vi "sqlread_write.vi"() -> ()   [LabVIEW 2017]
uses:
  <vilib>/addons/database/Connection.llb/DB Tools Open Connec (Path).vi
  <vilib>/addons/database/NI_Database_API.lvlib
panel:
  out "TRUE no barcode Done on station 1":bool
  out "FALSE healty":bool
  out "TRUE Duplication on Station 2":bool
  out "data":string[][](array[string])
  out "error out":errorcluster
  in  "error in (no error)":errorcluster
  # "testing vi"
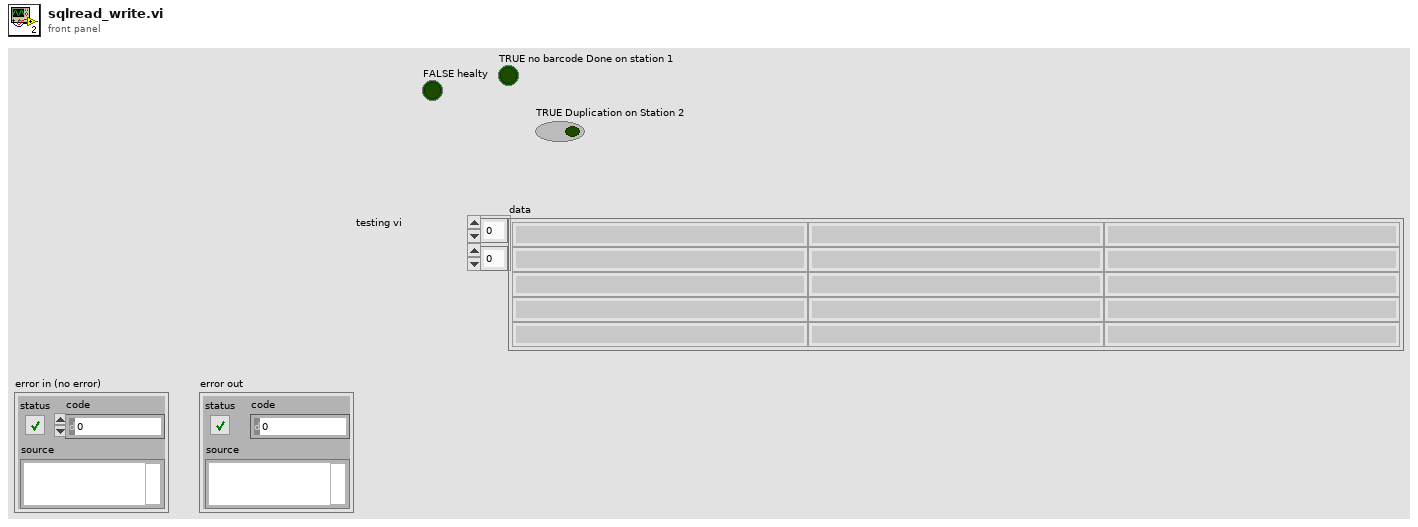
[diagram p1: front panel]
types:
  T1 = typedef "NI_Database_API.lvlib/Conn ObjectReference.ctl" = refnum<k1>
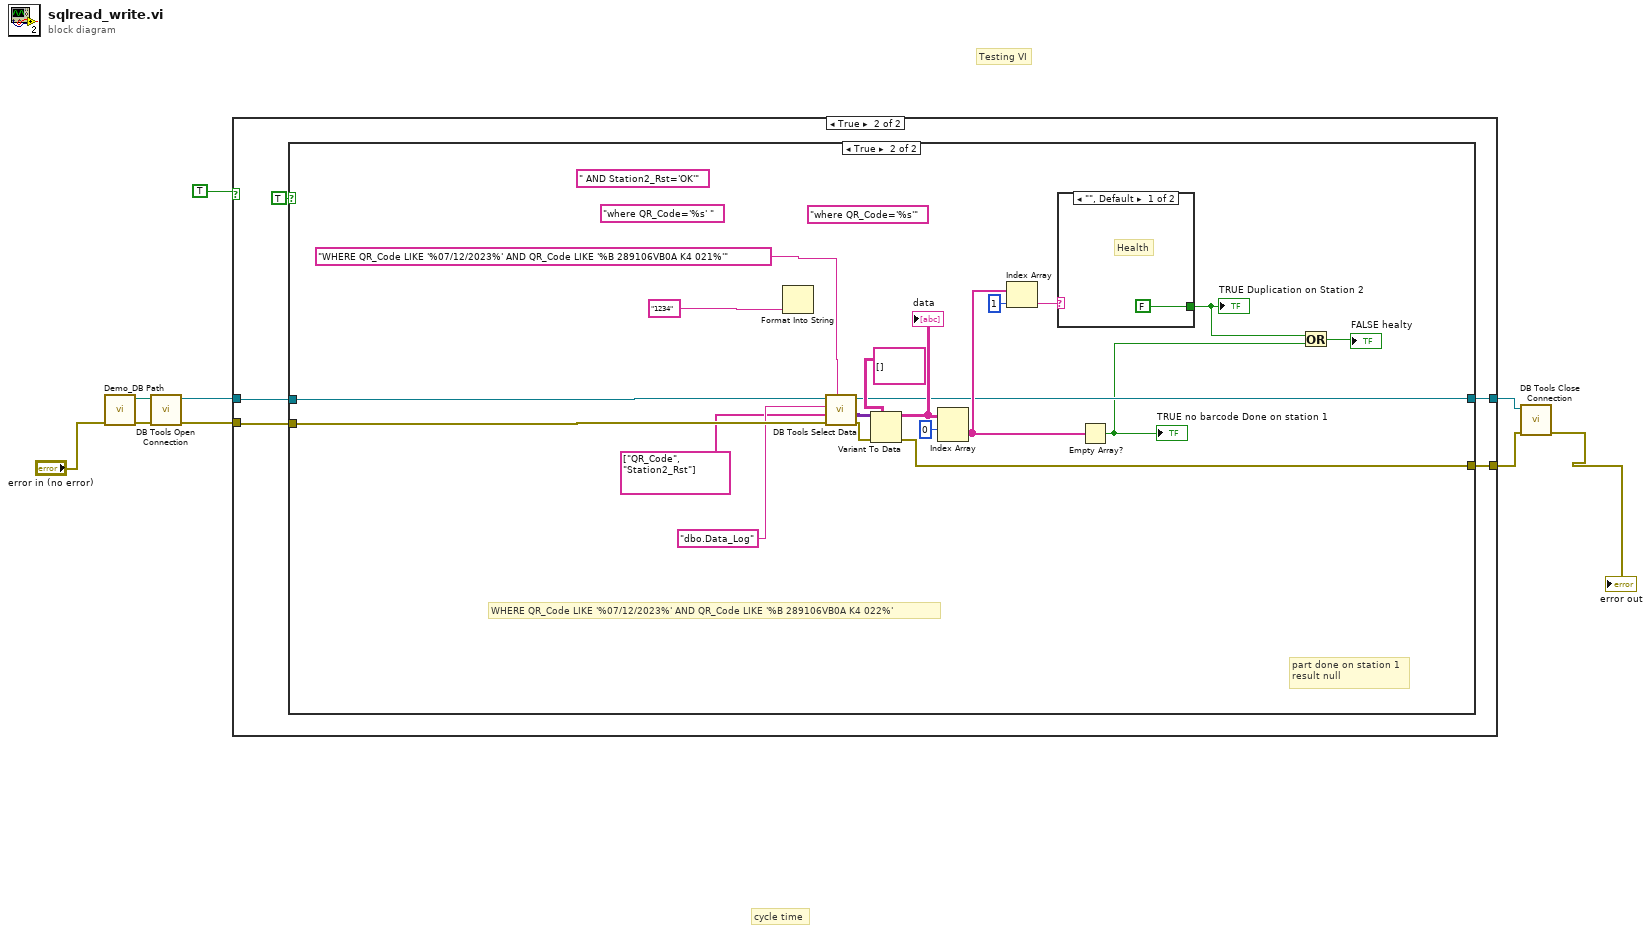
[diagram p0: block diagram]
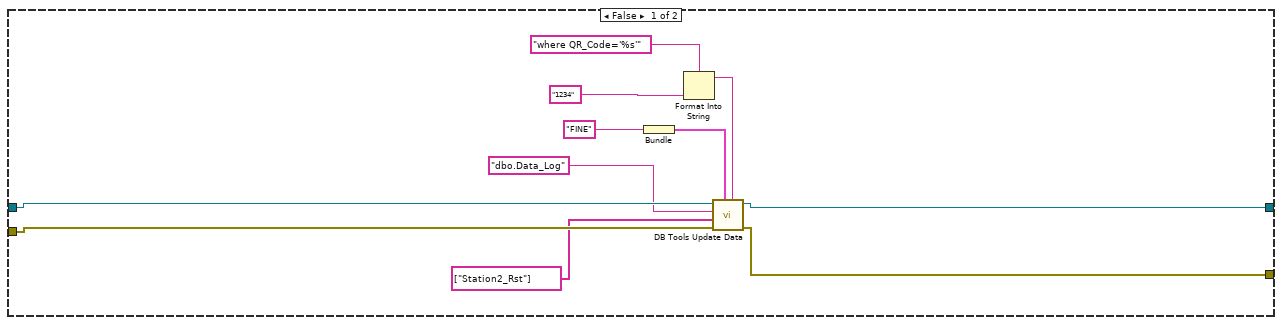
[diagram p2: hidden frame]
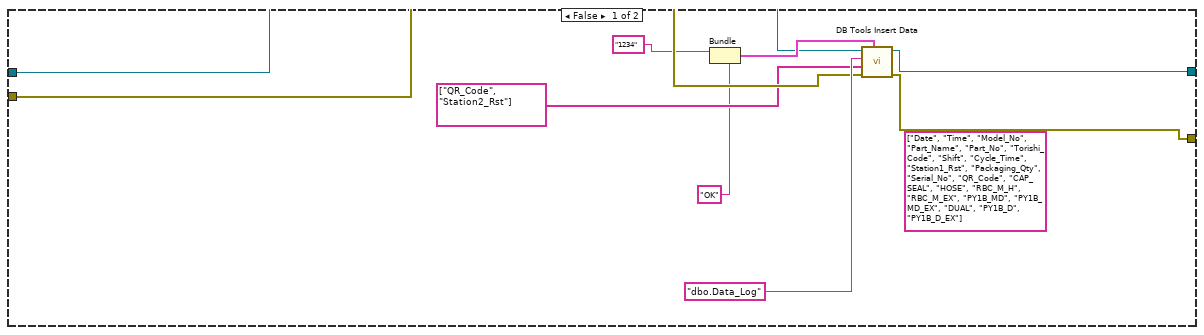
[diagram p3: hidden frame]
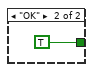
[diagram p4: hidden frame]
diagram:
  # "Testing VI"
  # "cycle time"
  n1 = call "Demo_DB Path.vi"("error in"="error in (no error)") -> ("error out"=w9:errorcluster, "DB Path"=w8:path)  [unwired: 9 in]
  n2 = call-poly <vilib>:"DB Tools Open Connection.vi"("error in (no error)"=w9, "connection information"=w8) -> ("error out"=w6:errorcluster, "connection reference"=w7:T1)  [unwired: 6 in]
  n3 = case shown="True" TRUE {
    tunnel: w7 -> [w18 w25]
    tunnel: w6 -> [w20 w24]
    tunnel: [w19 w23] -> w4
    tunnel: [w17 w22] -> w2
    frame False {
      n4 = Bundle("replace %s"="FINE") -> (w11:cluster{"replace %s":string})  [unwired: 1 in]
      n5 = Format Into String(format string="where QR_Code='%s'", "1234" ("replace %s")) -> (resulting string=w14:string)  [unwired: 2 in, 1 out]
      n6 = call <vilib>:"DB Tools Update Data.vi"("condition"=w14, "data"=w11, "error in (no error)"=w20, "columns"=string[] ["Station2_Rst"] ("columns 2"), "table"="dbo.Data_Log", "connection reference"=w18) -> ("error out"=w19:errorcluster, "connection reference out"=w17:T1)  [unwired: 4 in]
    }
    frame True {
      n7 = case shown="True" TRUE {
        tunnel: w25 -> [w29 w44]
        tunnel: w24 -> [w30 w43]
        tunnel: [w31 w42] -> w23
        tunnel: [w32 w41] -> w22
        frame False {
          (unwired) string[] ["Date", "Time", "Model_No", "Part_Name", "Part_No", "Torishi_Code", "Shift", "Cycle_Time", "Station1_Rst", "Packaging_Qty", "Serial_No", "QR_Code", "CAP_SEAL", "HOSE", "RBC_M_H", "RBC_M_EX", "PY1B_MD", "PY1B_MD_EX", "DUAL", "PY1B_D", "PY1B_D_EX"] ("columns 2")
          n8 = Bundle("table"="1234", "table"="OK") -> (w34:cluster{"table":string, "table":string})  [unwired: 1 in]
          n9 = call <vilib>:"DB Tools Insert Data.vi"("data"=w34, "error in (no error)"=w30, "columns"=string[] ["QR_Code", "Station2_Rst"] ("columns 2"), "table"="dbo.Data_Log", "connection reference"=w29) -> ("error out"=w31:errorcluster, "connection reference out"=w32:T1)  [unwired: 5 in]
        }
        frame True {
          (unwired) "where QR_Code='%s'" ("format string")
          (unwired) " AND Station2_Rst='OK'" ("replace %s")
          (unwired) "where QR_Code='%s' " ("format string")
          # "WHERE QR_Code LIKE '%07/12/2023%' AND QR_Code LIKE '%B 289106VB0A K4 022%'"
          # "part done on station 1\nresult null"
          n10 = Format Into String("1234" ("replace %s")) -> ()  [unwired: 3 in, 2 out]
          n11 = call <vilib>:"DB Tools Select Data.vi"("condition"="WHERE QR_Code LIKE '%07/12/2023%' AND QR_Code LIKE '%B 289106VB0A K4 021%'" ("format string"), "error in (no error)"=w43, "columns"=string[] ["QR_Code", "Station2_Rst"] ("columns 2"), "table"="dbo.Data_Log", "connection reference"=w44) -> ("error out"=w48:errorcluster, "data"=w50:variant[][], "connection reference out"=w41:T1)  [unwired: 1 in]
          n12 = Variant To Data(error in=w48, type=string[][] [], Variant=w50) -> (data=w49:string[][], error out=w42:errorcluster)
          "data" <- w49
          n13 = Index Array(array=w49, index (row)=0) -> (element=w46:string[])  [unwired: 1 in]
          n14 = Index Array(array=w46, index=1 ("index (row)")) -> (element=w45:string)
          n15 = case shown="\"\", Default" w45 {
            tunnel: [FALSE TRUE] -> w38
            frame "", Default {
              # "Health"
            }
            frame "OK" {
            }
          }
          "TRUE Duplication on Station 2" <- w38
          n16 = Empty Array?(array=w46) -> (empty?=w37:bool)
          "TRUE no barcode Done on station 1" <- w37
          n17 = Or(x=w38, y=w37) -> (x .or. y?=→"FALSE healty":bool)
        }
      }
    }
  }
  n18 = call <vilib>:"DB Tools Close Connection.vi"("error in (no error)"=w4, "connection reference"=w2) -> ("error out"=→"error out":errorcluster)  [unwired: 5 in]
